vi "Send ParametersUpdated.vi"(7 "Message Priority (Normal)":T2=enum."Normal", 8 "error in (no error)":errorcluster, 10 "Current Parameters":T1, 11 "Message Enqueuer":refnum<class "Message Enqueuer.lvclass">) -> (0 "error out":errorcluster, 3 "Message Enqueuer out":refnum<class "Message Enqueuer.lvclass">)   [LabVIEW 2023, in "Spectrometer Library.lvlib" / "SpectrometerComm.lvlib" / "ParametersUpdated Msg.lvclass"]
doc: "This VI sends the message to an actor."
uses:
  ParametersUpdated Msg.lvclass
  <vilib>/ActorFramework/Message Enqueuer/Message Enqueuer.lvclass
  <vilib>/ActorFramework/Message Enqueuer/Message Priority.ctl
  ParametersUpdated Msg.lvclass/ParametersUpdated Msg.ctl
  <vilib>/ActorFramework/Message Enqueuer/Message Enqueuer.lvclass/Message Enqueuer.ctl
  <vilib>/ActorFramework/Message Priority Queue/Priority Enqueue.vi
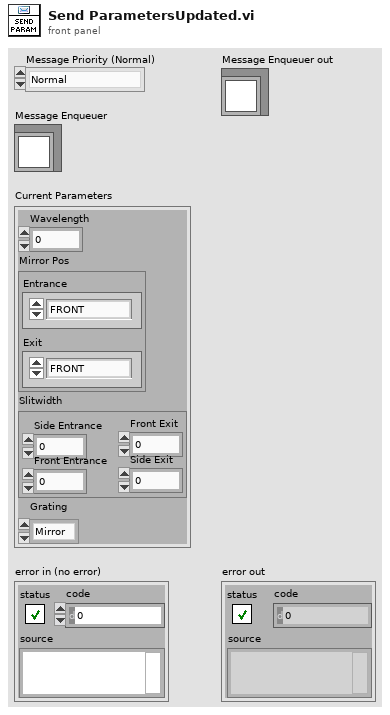
[diagram p1: front panel]
types:
  T1 = cluster{"Wavelength":dbl, "Mirror Pos":cluster{"Entrance":enum16{"FRONT", "SIDE"}, "Exit":enum16{"FRONT", "SIDE"}}, "Slitwidth":cluster{"Side Entrance":u16, "Front Entrance":u16, "Front Exit":u16, "Side Exit":u16}, "Grating":enum16{"Mirror", "1200 g/mm", "1800 g/mm"}}
  T2 = typedef "Actor Framework.lvlib/Message Enqueuer.lvclass/Message Priority.ctl" = enum16{"Low", "Normal", "High"}
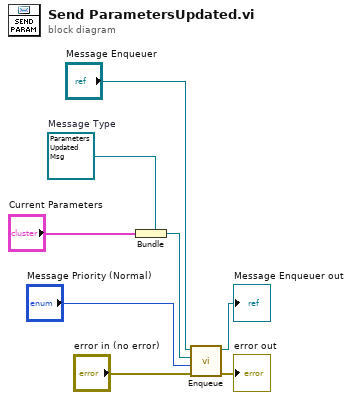
[diagram p0: block diagram]
diagram:
  w5 = refnum<class "ParametersUpdated Msg.lvclass"> refnum  # Message Type
  n1 = Bundle(cluster=w5, "Current Parameters") -> (w4:refnum<class "ParametersUpdated Msg.lvclass">)
  n2 = call <vilib>:"Enqueue.vi"("error in (no error)"="error in (no error)", "Message Priority (Normal)"="Message Priority (Normal)", "Message"=w4, "Message Enqueuer in"="Message Enqueuer") -> ("error out"=→"error out":errorcluster, "Message Enqueuer out"=→"Message Enqueuer out":refnum<class "Message Enqueuer.lvclass">)  [unwired: 6 in]
